vi "Convert to JSON Comp Format.vi"(11 "digital audio protocol settings":T2={"number of channels"=0, "data justification"=enum."Left Justified", "endianness"=enum."LSB First", "channel length"=0, "bit depth"=0, "frame clock rate"=0.0, "bit clock edge sync"=enum."Falling", "master clock rate"=0.0, "Logic Level"=enum."1.2 V", "frame sync edge for channel 0"=enum."Rising", "Channel 0 Offset"=0}) -> (3 "JSON compatible settings":T1)   [LabVIEW 2023, in "digital audio protocol controls.lvlib"]
uses:
  digital audio protocol controls.lvlib
  controls/digital serial gen settings.ctl
  <vilib>/PDM Acquisition Toolkit/shared/controls/PCM Data Justification.ctl
  <vilib>/PDM Acquisition Toolkit/shared/controls/PCM Bit Endianness.ctl
  <vilib>/PDM Acquisition Toolkit/shared/controls/Digital Edge.ctl
  <vilib>/PDM Acquisition Toolkit/host/Classes/Session/Controls/Logic Levels.ctl
  digital serial gen settings_json.ctl
  <vilib>/PDM Acquisition Toolkit/shared/PDM Shared.lvlib
  <vilib>/PDM Acquisition Toolkit/host/Classes/Session/DecoderSession.lvclass
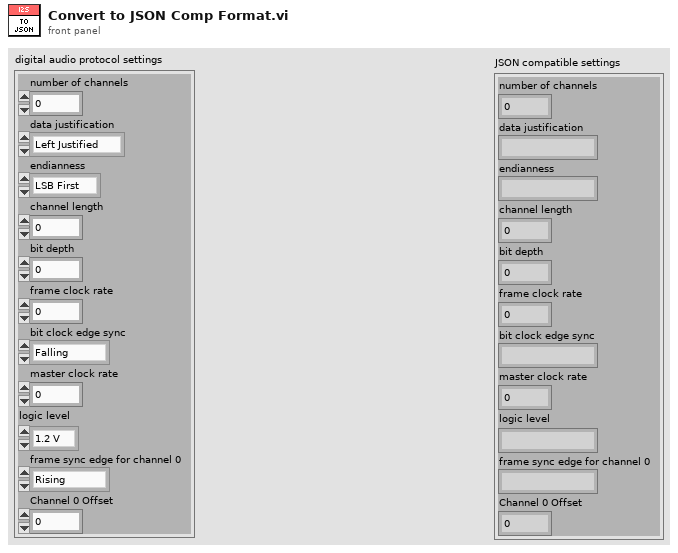
[diagram p1: front panel]
types:
  T1 = typedef "digital audio protocol controls.lvlib/digital serial gen settings_json.ctl" = cluster{"number of channels":u32, "data justification":string, "endianness":string, "channel length":u32, "bit depth":u32, "frame clock rate":dbl, "bit clock edge sync":string, "master clock rate":dbl, "logic level":string, "frame sync edge for channel 0":string, "Channel 0 Offset":u32}
  T2 = typedef "digital serial gen settings.ctl" = cluster{"number of channels":u32, "data justification":T3, "endianness":T4, "channel length":u32, "bit depth":u32, "frame clock rate":dbl, "bit clock edge sync":T5, "master clock rate":dbl, "Logic Level":T6, "frame sync edge for channel 0":T5, "Channel 0 Offset":u32}
  T3 = typedef "PDM Shared.lvlib/PCM Data Justification.ctl" = enum16{"Left Justified", "Right Justified"}
  T4 = typedef "PDM Shared.lvlib/PCM Bit Endianness.ctl" = enum16{"MSB First", "LSB First"}
  T5 = typedef "PDM Shared.lvlib/Digital Edge.ctl" = enum8{"Rising", "Falling"}
  T6 = typedef "PDM Acquisition Class Library.lvlib/DecoderSession.lvclass/Logic Levels.ctl" = enum16{"3.3 V", "1.8 V", "1.2 V"}
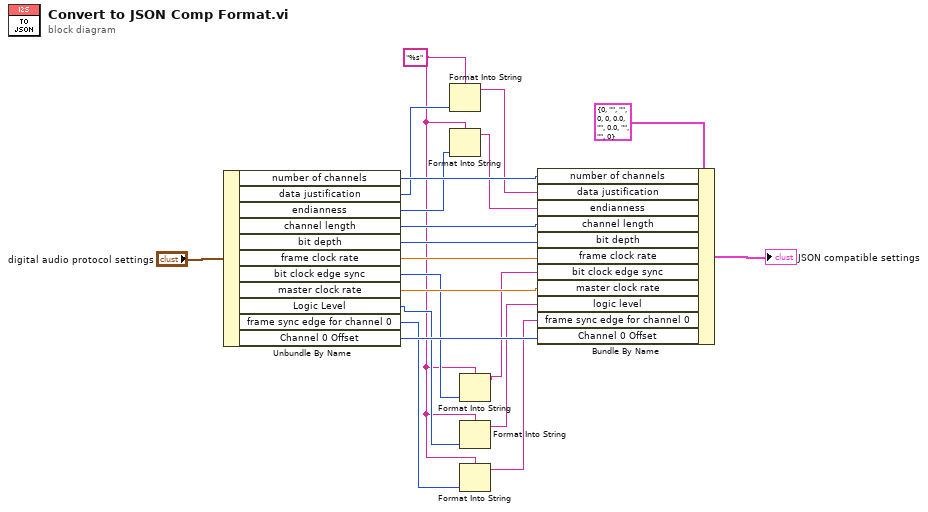
[diagram p0: block diagram]
diagram:
  w1 = "%s" ("format string")
  n1 = Unbundle By Name("digital audio protocol settings") -> ("number of channels"=w17:u32, "data justification"=w11:T3, "endianness"=w9:T4, "channel length"=w16:u32, "bit depth"=w15:u32, "frame clock rate"=w14:dbl, "bit clock edge sync"=w7:T5, "master clock rate"=w13:dbl, "Logic Level"=w6:T6, "frame sync edge for channel 0"=w5:T5, "Channel 0 Offset"=w12:u32)
  n2 = Format Into String(format string=w1, w11) -> (resulting string=w10:string)  [unwired: 2 in, 1 out]
  n3 = Format Into String(format string=w1, w9) -> (resulting string=w8:string)  [unwired: 2 in, 1 out]
  n4 = Format Into String(format string=w1, w7) -> (resulting string=w3:string)  [unwired: 2 in, 1 out]
  n5 = Format Into String(format string=w1, w6) -> (resulting string=w2:string)  [unwired: 2 in, 1 out]
  n6 = Format Into String(format string=w1, w5) -> (resulting string=w4:string)  [unwired: 2 in, 1 out]
  n7 = Bundle By Name(cluster=T1 {"number of channels"=0, "data justification"="", "endianness"="", "channel length"=0, "bit depth"=0, "frame clock rate"=0.0, "bit clock edge sync"="", "master clock rate"=0.0, "logic level"="", "frame sync edge for channel 0"="", "Channel 0 Offset"=0} ("JSON compatible settings"), "number of channels"=w17, "data justification"=w10, "endianness"=w8, "channel length"=w16, "bit depth"=w15, "frame clock rate"=w14, "bit clock edge sync"=w3, "master clock rate"=w13, "logic level"=w2, "frame sync edge for channel 0"=w4, "Channel 0 Offset"=w12) -> (→"JSON compatible settings":T1)
